vi "FindClosestPreset.vi"(11 "output cluster":T1) -> (1 "corrected Height":dbl, 2 "ClosestPresetIndex":dbl, 3 "CurrentPosition":dbl)   [LabVIEW 2014]
uses:
  buttons/PresetValues.ctl
  <vilib>/Rock Robotics/Network Tables/SD Read Number.vi
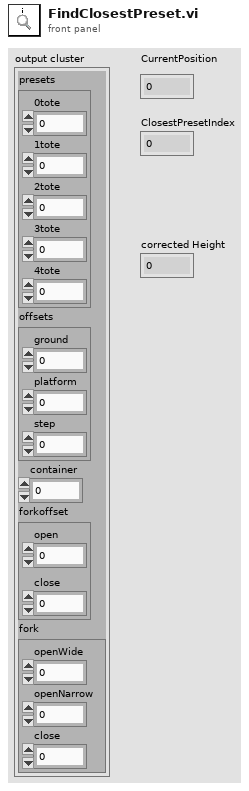
[diagram p1: front panel]
types:
  T1 = typedef "PresetValues.ctl" = cluster{"presets":cluster{"0tote":dbl, "1tote":dbl, "2tote":dbl, "3tote":dbl, "4tote":dbl}, "offsets":cluster{"ground":dbl, "platform":dbl, "step":dbl}, "container":dbl, "forkoffset":cluster{"open":dbl, "close":dbl}, "fork":cluster{"openWide":dbl, "openNarrow":dbl, "close":dbl}}
  T2 = cluster{"0tote":dbl, "1tote":dbl, "2tote":dbl, "3tote":dbl, "4tote":dbl}
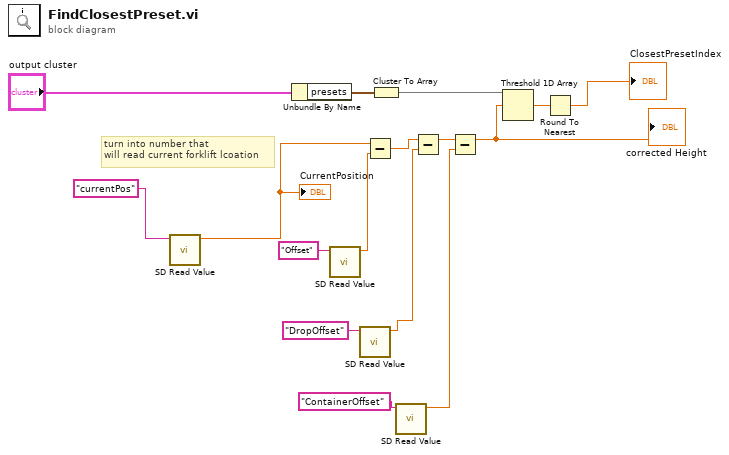
[diagram p0: block diagram]
diagram:
  # "turn into number that\nwill read current forklift lcoation"
  n1 = call-poly <vilib>:"SD Read Value.vi"("Name"="currentPos") -> ("Numeric"=w6:dbl)  [unwired: 8 in, 2 out]
  "CurrentPosition" <- w6
  n2 = Unbundle By Name("output cluster") -> ("presets"=w2:T2)
  n3 = call-poly <vilib>:"SD Read Value.vi"("Name"="Offset") -> ("Numeric"=w7:dbl)  [unwired: 8 in, 2 out]
  n4 = call-poly <vilib>:"SD Read Value.vi"("Name"="DropOffset") -> ("Numeric"=w13:dbl)  [unwired: 8 in, 2 out]
  n5 = Subtract(x=w6, y=w7) -> (x-y=w5:dbl)
  n6 = Cluster To Array(cluster=w2) -> (array=w4:dbl[])
  n7 = call-poly <vilib>:"SD Read Value.vi"("Name"="ContainerOffset") -> ("Numeric"=w15:dbl)  [unwired: 8 in, 2 out]
  n8 = Subtract(x=w5, y=w13) -> (x-y=w12:dbl)
  n9 = Subtract(x=w12, y=w15) -> (x-y=w14:dbl)
  "corrected Height" <- w14
  n10 = Threshold 1D Array(2:w14, 3:w4) -> (0:w16:dbl)  [unwired: 1 in]
  n11 = Round To Nearest(number=w16) -> (nearest integer value=→"ClosestPresetIndex":dbl)
